vi "LVClass_Image get image information.vi"(0 "Image in":refnum<class "Image.lvclass">, 11 "error in (no error)":errorcluster) -> (4 "Image out":refnum<class "Image.lvclass">, 6 "Acquisition information":T1={"Image general information"={"Camera serial number"="", "Smearing removed"=FALSE, "Background image removed"=FALSE, "Time Stamp"=timestamp(0 s since 1904-01-01), "Comment"="", "Camera_MAX_Level"=0}, "Acquisition information"={"Exposure duration (us)"=0, "Exposure duration specified (us)"=0, "Gain"=0.0, "Number of summed images"=0, "Trigger type"=""}, "Number of pixels"={"X"=0, "Y"=0}, "Number of bits"=enum."16"}, 15 "error out":errorcluster)   [LabVIEW 2020, in "Image.lvclass"]
doc: "Get metadata from Image object.\n\n--------------------------------------------------------------------------------\n\n<B>ImageIn </B> : Image object.\n<B>ImageOut </B> : Image object.\n<B>haso_serial_number </B> : Haso serial number.\n<B>camera_serial_number </B> : Camera serial number.\n<B>exposure_time_applied </B> : Exposure duration applied (us).\n<B>exposure_time_requested </B> : Exposure duration requested (us).\n<B>gain </B> : Applied gain (SI).\n<B>nb_summed_images </B> : Number of summed images.\n<B>is_smearing_removed </B> : Smearing_removed.\n<B>is_background_removed </B> : Background_removed.\n<B>trigger_type </B> : Trigger mode.\n<B>time_stamp </B> : Date of the acquired Image.\n<B>max_level </B> : Max level value.\n<B>comments </B> : Comments.\n<B>ErrorIn </B> : Error\n<B>ErrorOut </B> : Error\n\n--------------------------------------------------------------------------------"
uses:
  Image.lvclass
  Controls/Image information.ctl
  Controls/Image general information.ctl
  Controls/Image acquisition information.ctl
  Controls/Point2D.ctl
  Controls/Data alignment enum.ctl
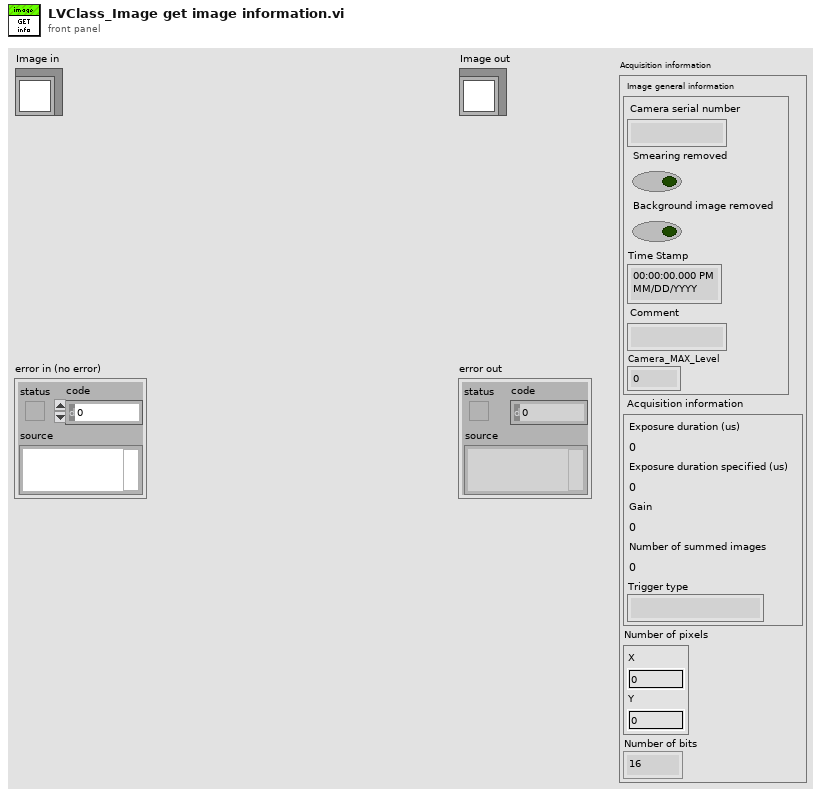
[diagram p1: front panel]
types:
  T1 = typedef "Image information.ctl" = cluster{"Image general information":T2, "Acquisition information":T3, "Number of pixels":T4, "Number of bits":T5}
  T2 = typedef "Image general information.ctl" = cluster{"Camera serial number":string, "Smearing removed":bool, "Background image removed":bool, "Time Stamp":timestamp, "Comment":string, "Camera_MAX_Level":i32}
  T3 = typedef "Image acquisition information.ctl" = cluster{"Exposure duration (us)":i32, "Exposure duration specified (us)":i32, "Gain":sgl, "Number of summed images":i32, "Trigger type":string}
  T4 = typedef "Point2D.ctl" = cluster{"X":u32, "Y":u32}
  T5 = typedef "Data alignment enum.ctl" = enum16{"8", "16", "32"}
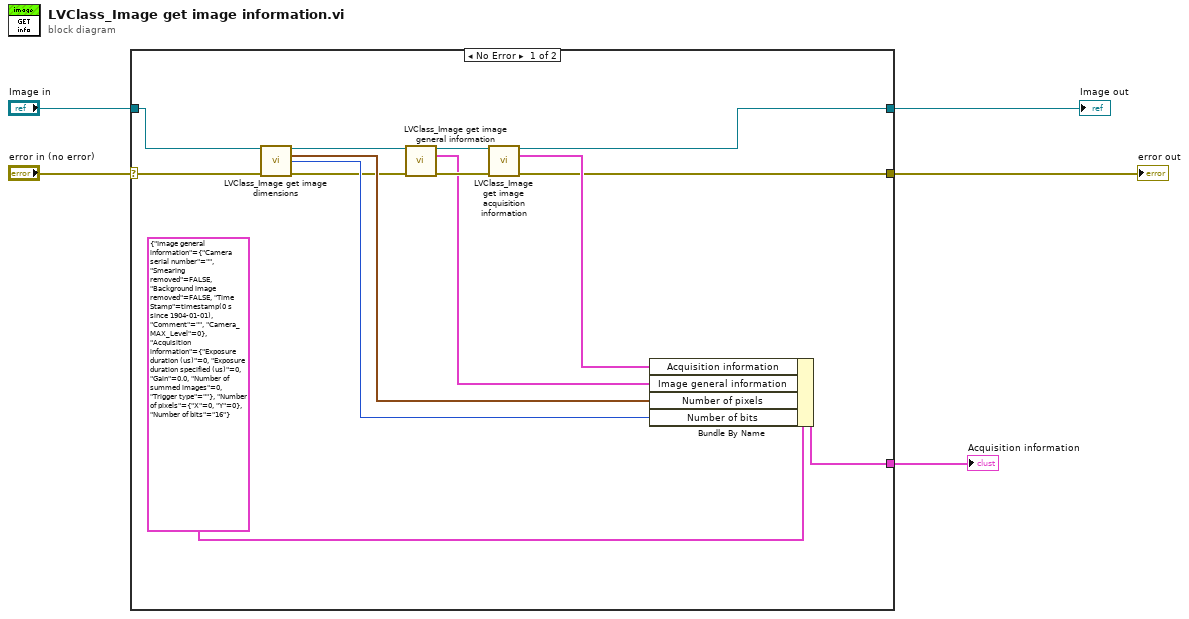
[diagram p0: block diagram]
diagram:
  n1 = case shown="No Error" "error in (no error)" {
    selector: "error in (no error)" -> [w17 w21]
    tunnel: [w6 w21] -> w4
    tunnel: [w7 w20] -> w2
    tunnel: "Image in" -> [w18 w20]
    tunnel: [w19 _] -> w1
    frame No Error {
      n2 = call "LVClass_Image get image dimensions.vi"("Image in"=w18, "error in (no error)"=w17) -> ("Image out"=w8:refnum<class "Image.lvclass">, "Number of pixels"=w15:T4, "Number of bits"=w14:T5, "error out"=w13:errorcluster)  [unwired: 10 in]
      n3 = call "LVClass_Image get image general information.vi"("Image in"=w8, "error in (no error)"=w13) -> ("Image out"=w12:refnum<class "Image.lvclass">, "Acquisition information"=w9:T2, "error out"=w11:errorcluster)  [unwired: 11 in]
      n4 = call "LVClass_Image get image acquisition information.vi"("Image in"=w12, "error in (no error)"=w11) -> ("Image out"=w7:refnum<class "Image.lvclass">, "Acquisition information"=w10:T3, "error out"=w6:errorcluster)  [unwired: 11 in]
      n5 = Bundle By Name(cluster=T1 {"Image general information"={"Camera serial number"="", "Smearing removed"=FALSE, "Background image removed"=FALSE, "Time Stamp"=timestamp(0 s since 1904-01-01), "Comment"="", "Camera_MAX_Level"=0}, "Acquisition information"={"Exposure duration (us)"=0, "Exposure duration specified (us)"=0, "Gain"=0.0, "Number of summed images"=0, "Trigger type"=""}, "Number of pixels"={"X"=0, "Y"=0}, "Number of bits"=enum."16"} ("Acquisition information"), "Acquisition information"=w10, "Image general information"=w9, "Number of pixels"=w15, "Number of bits"=w14) -> (w19:T1)
    }
    frame Error {
    }
  }
  "error out" <- w4
  "Image out" <- w2
  "Acquisition information" <- w1
